vi "Reset NIC.vi"(8 "Error In":errorcluster, 10 "NIC Name":string, 11 "Install LV Data":T1) -> (0 "Error Out":errorcluster, 3 "Install LV Data out":T1)   [LabVIEW 2014, in "LMH-LINX.lvlib"]
uses:
  <vilib>/MakerHub/LINX/LMH-LINX.lvlib
  <vilib>/MakerHub/LINX/Private/Utilties/Target Management/Install LV Data.ctl
  C:/Program Files (x86)/National Instruments/LabVIEW 2014/vi.lib/MakerHub/LINX/Resources/Renci.SshNet.dll
  Resources/Renci.SshNet.dll
  <vilib>/MakerHub/LINX/Private/Utilties/Target Management/Target Info.ctl
  <vilib>/MakerHub/LINX/Private/Utilties/Target Management/NIC Info.ctl
  <vilib>/MakerHub/LINX/Private/Utilties/Target Management/NIC Mode.ctl
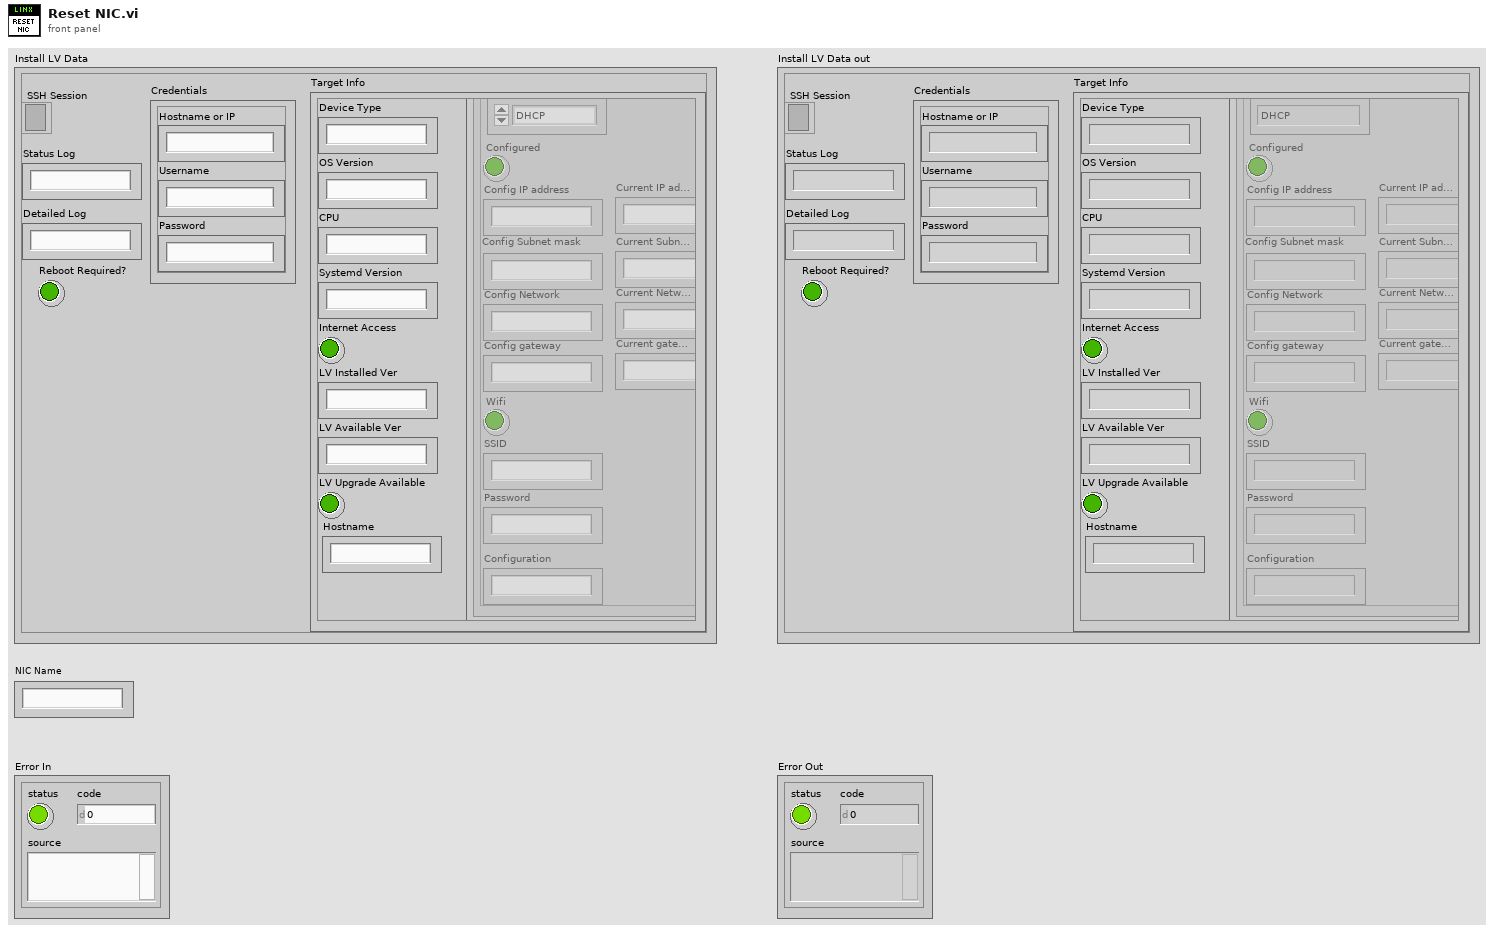
[diagram p1: front panel]
types:
  T1 = typedef "LMH-LINX.lvlib/Install LV Data.ctl" = cluster{"SSH Session":refnum<k24>, "Status Log":string, "Detailed Log":string, "Credentials":cluster{"Hostname or IP":string, "Username":string, "Password":string}, "Target Info":T2, "Reboot Required?":bool}
  T2 = typedef "LMH-LINX.lvlib/Target Info.ctl" = cluster{"OS Version":string, "CPU":string, "Systemd Version":string, "Internet Access":bool, "Device Type":string, "LV Installed Ver":string, "LV Available Ver":string, "LV Upgrade Available":bool, "Hostname":string, "NIC Info":T3[]}
  T3 = typedef "LMH-LINX.lvlib/NIC Info.ctl" = cluster{"Name":string, "NIC Mode":T4, "Configured":bool, "Config IP address":string, "Config Subnet mask":string, "Config Network":string, "Config gateway":string, "Wifi":bool, "SSID":string, "Password":string, "Configuration":string, "Current IP address":string, "Current Subnet mask":string, "Current gateway":string, "Current Network":string}
  T4 = typedef "LMH-LINX.lvlib/NIC Mode.ctl" = enum16{"DHCP", "Static", "Loopback"}
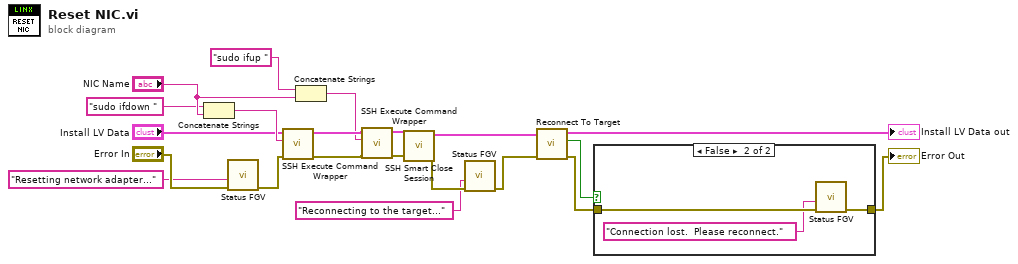
[diagram p0: block diagram]
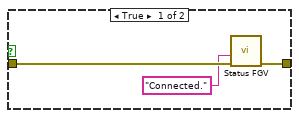
[diagram p2: hidden frame]
diagram:
  n1 = Concatenate Strings("sudo ifdown " ("string"), "NIC Name") -> (w20:string)
  n2 = call <vilib>:"Status FGV.vi"("Error In"="Error In", "Status"="Resetting network adapter...") -> ("Error Out"=w14:errorcluster)  [unwired: 7 in, 2 out]
  n3 = call <vilib>:"SSH Execute Command Wrapper.vi"("Error In"=w14, "Command"=w20, "Install LV Data in"="Install LV Data") -> ("Error Out"=w3:errorcluster, "Install LV Data out"=w2:T1)  [unwired: 6 in, 1 out]
  n4 = Concatenate Strings("sudo ifup " ("string"), "NIC Name") -> (w1:string)
  n5 = call <vilib>:"SSH Execute Command Wrapper.vi"("Error In"=w3, "Command"=w1, "Install LV Data in"=w2) -> ("Error Out"=w4:errorcluster, "Install LV Data out"=w5:T1)  [unwired: 6 in, 1 out]
  n6 = call <vilib>:"SSH Smart Close Session.vi"("Error In"=w4, "Install LV Data"=w5) -> ("Error Out"=w12:errorcluster, "Install LV Data"=w11:T1)  [unwired: 8 in]
  n7 = call <vilib>:"Status FGV.vi"("Error In"=w12, "Status"="Reconnecting to the target...") -> ("Error Out"=w10:errorcluster)  [unwired: 7 in, 2 out]
  n8 = call <vilib>:"Reconnect To Target.vi"("Error In"=w10, "Install LV Data in"=w11) -> ("Error Out"=w8:errorcluster, "Connected?"=w6:bool, "Install LV Data out"=→"Install LV Data out":T1)  [unwired: 7 in]
  n9 = case shown="False" w6 {
    tunnel: w8 -> [w24 w27]
    tunnel: [w23 w26] -> w7
    frame True {
      n10 = call <vilib>:"Status FGV.vi"("Error In"=w24, "Status"="Connected.") -> ("Error Out"=w23:errorcluster)  [unwired: 7 in, 2 out]
    }
    frame False {
      n11 = call <vilib>:"Status FGV.vi"("Error In"=w27, "Status"="Connection lost.  Please reconnect.") -> ("Error Out"=w26:errorcluster)  [unwired: 7 in, 2 out]
    }
  }
  "Error Out" <- w7
